vi "Minify.vi"(4 "Disable LabVIEW Extensions":bool, 8 "error in (no error)":errorcluster, 10 "Offset":i32, 11 "JSON":string) -> (0 "error out":errorcluster, 2 "Rest of Input String":string, 3 "<JSON>":string caption="<JSON>First JSON Value")   [LabVIEW 2021, in "json.facade.lvlib"]
doc: "\"Minify\" a JSON Value, removing all whitespace (and stripping any comments)."
uses:
  json.facade.lvlib
  jsontext/JSONtext.lvlib
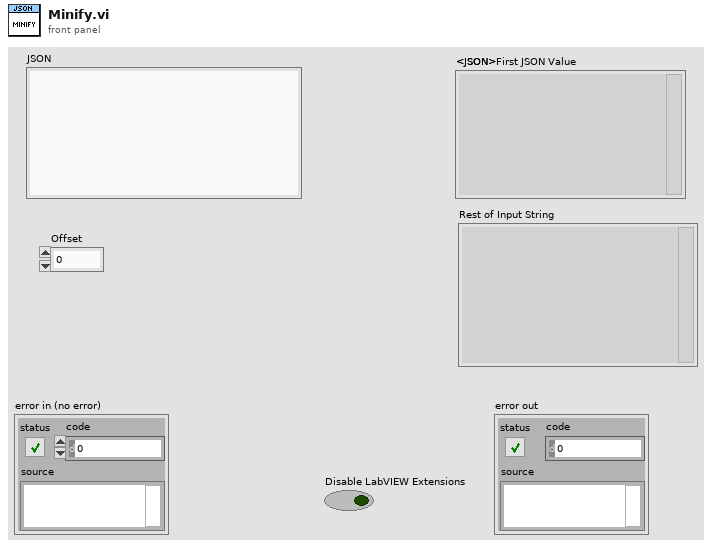
[diagram p1: front panel]
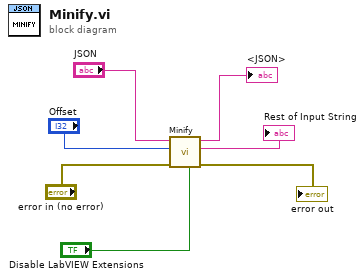
[diagram p0: block diagram]
diagram:
  n1 = call "Minify.vi"("Disable LabVIEW Extensions"="Disable LabVIEW Extensions", "error in (no error)"="error in (no error)", "Offset"="Offset", "JSON"="JSON") -> ("error out"=→"error out":errorcluster, "Rest of Input String"=→"Rest of Input String":string, "<JSON>"=→"<JSON>":string)  [unwired: 5 in]
